vi "Do Calculation.vi"(8 "error in (no error)":errorcluster, 11 "CPU FFT Calculator in":refnum<class "CPU FFT Calculator.lvclass">) -> (0 "error out":errorcluster, 3 "CPU FFT Calculator out":refnum<class "CPU FFT Calculator.lvclass">)   [LabVIEW 2020, in "CPU FFT Calculator.lvlib" / "CPU FFT Calculator.lvclass"]
uses:
  CPU FFT Calculator.lvclass
  C:/Users/natan/Documents/G2CPU-Performance-Demo/Calculation Worker/Calculation Worker/Calculation Worker.lvclass
  C:/Program Files/National Instruments/LabVIEW 2026/vi.lib/ActorFramework/Actor/Actor.lvclass
  CPU FFT Calculator.lvclass/CPU FFT Calculator.ctl
  CPU Calculation Results.ctl
  <vilib>/ActorFramework/Actor/Actor.lvclass/Actor.ctl
  <vilib>/ActorFramework/Message Enqueuer/Message Enqueuer.lvclass/Message Enqueuer.ctl
  CPU FFT Calculator Messages/Process Calculation Results Msg/Process Calculation Results Msg.lvclass/Process Calculation Results Msg.ctl
  <vilib>/Analysis/2dsp.llb/Complex FFT.vi
  <vilib>/ActorFramework/Message Enqueuer/Init from Existing Queue.vi
  <vilib>/ActorFramework/Message Enqueuer/Enqueue.vi
  CPU FFT Calculator Messages/Process Calculation Results Msg/Process Calculation Results Msg.lvclass
  C:/Program Files/National Instruments/LabVIEW 2026/vi.lib/ActorFramework/Message/Message.lvclass
  CPU FFT Calculator Messages/Do Calculation Msg/Do Calculation Msg.lvclass
  CPU FFT Calculator Messages/Stop Calculation Msg/Stop Calculation Msg.lvclass
  <vilib>/ActorFramework/Message Priority Queue/Priority Enqueue.vi
  <vilib>/ActorFramework/Message Enqueuer/Message Enqueuer.lvclass
  <vilib>/Analysis/NI_AALPro.lvlib
  <vilib>/ActorFramework/Actor/Actor.lvclass
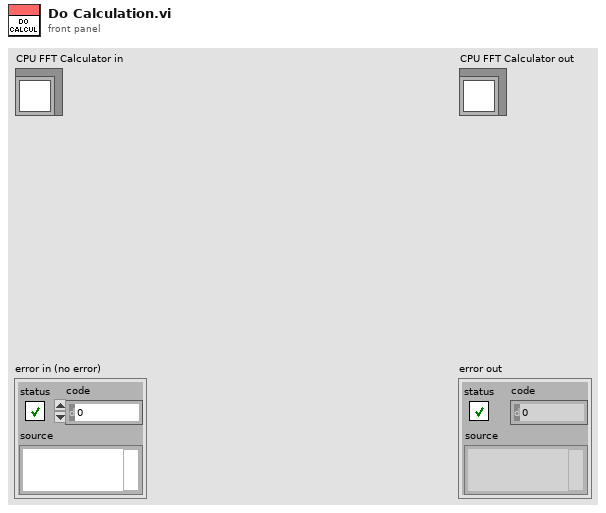
[diagram p1: front panel]
types:
  T1 = typedef "CPU FFT Calculator.lvlib/CPU FFT Calculator.lvclass/CPU Calculation Results.ctl" = cluster{"Result Array":sgl[], "Throughput Time":dbl, "FFT Time":dbl, "Buffer Size":i32}
  T2 = typedef "Data Source.lvlib/Data Source.lvclass/Data Source Buffer.ctl" = refnum<data-value>
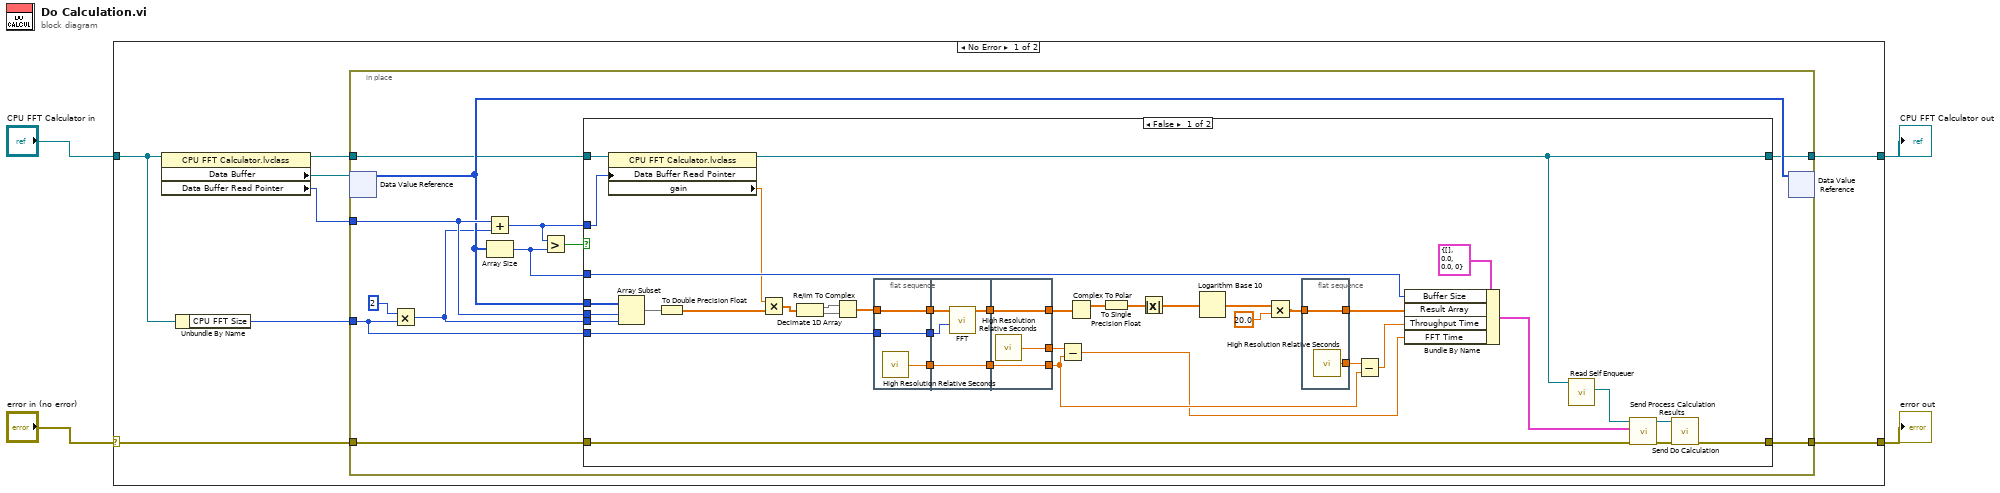
[diagram p0: block diagram]
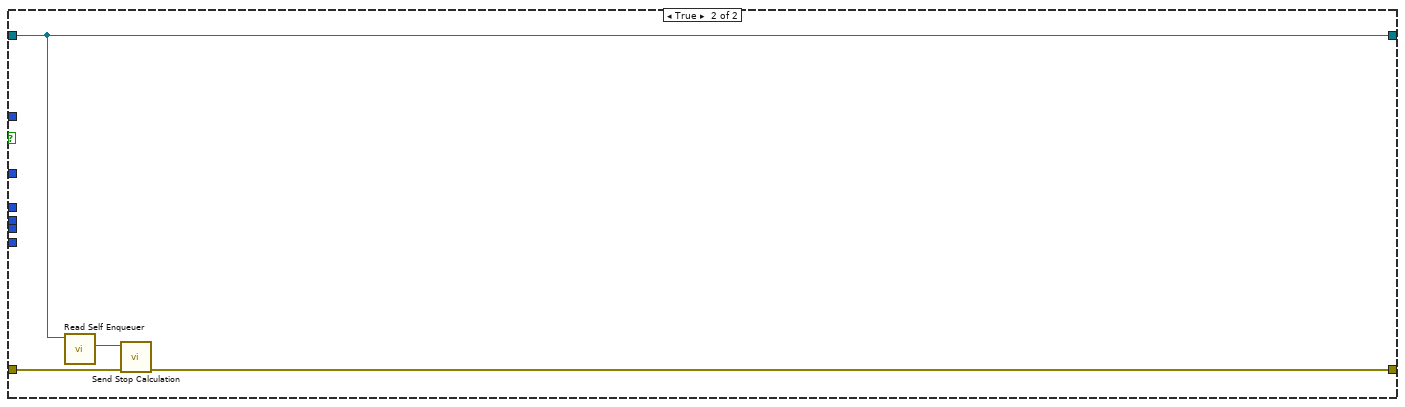
[diagram p2: hidden frame]
diagram:
  n1 = case shown="No Error" "error in (no error)" {
    selector: "error in (no error)" -> [w8 w82]
    tunnel: [w7 w82] -> w3
    tunnel: [w5 w81] -> w1
    tunnel: "CPU FFT Calculator in" -> [w12 w81]
    frame No Error {
      n2 = property class="CPU FFT Calculator.lvclass"(reference=w12) -> (reference out=w6:refnum<class "CPU FFT Calculator.lvclass">, "Data Buffer"=w11:T2, "Data Buffer Read Pointer"=w9:u64)  [unwired: 1 in, 1 out]
      n3 = Unbundle By Name(w12) -> ("CPU FFT Size"=w10:u64)
      n4 = in-place {
        in-place-border: w10 -> [w15]
        in-place-border: w9 -> [w24]
        in-place-border: w8 -> [w22]
        in-place-border: [w20] -> w7
        in-place-border: w6 -> [w19]
        in-place-border: [w17] -> w5
        n5 = in-place-dvr #1(w11) -> (w23:i16[])  [unwired: 1 out]
        n6 = Multiply(x=u64 2, y=w15) -> (x*y=w14:u64)
        n7 = Add(x=w24, y=w14) -> (x+y=w18:u64)
        n8 = Array Size(array=w23) -> (size(s)=w16:i32)
        n9 = Greater?(x=w18, y=w16) -> (0:w21:bool)
        n10 = case shown="False" w21 {
          tunnel: w24 -> [w51 _]
          tunnel: w14 -> [w50 _]
          tunnel: w23 -> [w46 _]
          tunnel: w22 -> [w38 w80]
          tunnel: [w37 w79] -> w20
          tunnel: w19 -> [w35 w77]
          tunnel: w18 -> [w34 _]
          tunnel: [w33 w77] -> w17
          tunnel: w16 -> [w32 _]
          tunnel: w15 -> [w31 _]
          frame False {
            n11 = property class="CPU FFT Calculator.lvclass"(reference=w35, "Data Buffer Read Pointer"=w34) -> (reference out=w33:refnum<class "CPU FFT Calculator.lvclass">, "gain"=w25:dbl)  [unwired: 1 in, 1 out]
            n12 = Array Subset(array=w46, index=w51, length=w50) -> (w53:i16[])
            n13 = To Double Precision Float(number=w53) -> (double precision float=w30:dbl[])
            n14 = Multiply(x=w25, y=w30) -> (x*y=w26:dbl[])
            n15 = Decimate 1D Array(w26) -> (w29:dbl[], w28:dbl[])
            n16 = Re/Im To Complex(1:w28, 2:w29) -> (0:w27:cdb[])
            n17 = flat-sequence {
              tunnel: w31 -> [w68]
              tunnel: w27 -> [w69]
              tunnel: [w69] -> w64
              tunnel: [w68] -> w63
              tunnel: [w67] -> w62
              tunnel: [w73] -> w61
              tunnel: w64 -> [w72]
              tunnel: w63 -> [w71]
              tunnel: w62 -> [w70]
              tunnel: [w70] -> w60
              tunnel: [w76] -> w54
              tunnel: w61 -> [w76]
              tunnel: [w75] -> w52
              tunnel: w60 -> [w74]
              tunnel: [w74] -> w47
              frame #0 {
                n18 = call <vilib>:"High Resolution Relative Seconds.vi"() -> ("relative seconds"=w67:dbl)
              }
              frame #1 {
                n19 = call-poly <vilib>:"FFT.vi"("FFT size"=w71, "X"=w72) -> ("FFT {X}"=w73:cdb[])  [unwired: 8 in, 1 out]
              }
              frame #2 {
                n20 = call <vilib>:"High Resolution Relative Seconds.vi"() -> ("relative seconds"=w75:dbl)
              }
            }
            n21 = Subtract(x=w52, y=w47) -> (x-y=w39:dbl)
            n22 = Complex To Polar(r * e^(i*theta)=w54) -> (r=w55:dbl[])  [unwired: 1 out]
            n23 = To Single Precision Float(number=w55) -> (single precision float=w56:sgl[])
            n24 = Absolute Value(x=w56) -> (abs(x)=w59:sgl[])
            n25 = Logarithm Base 10(1:w59) -> (0:w58:sgl[])
            n26 = Multiply(x=w58, y=sgl 20.0) -> (x*y=w49:sgl[])
            n27 = flat-sequence {
              tunnel: [w66] -> w41
              tunnel: w49 -> [w66]
              tunnel: [w65] -> w48
              frame #0 {
                n28 = call <vilib>:"High Resolution Relative Seconds.vi"() -> ("relative seconds"=w65:dbl)
              }
            }
            n29 = Subtract(x=w48, y=w47) -> (x-y=w40:dbl)
            n30 = Bundle By Name(cluster=T1 {"Result Array"=[], "Throughput Time"=0.0, "FFT Time"=0.0, "Buffer Size"=0} ("Calculation Results"), "Buffer Size"=w32, "Result Array"=w41, "Throughput Time"=w40, "FFT Time"=w39) -> (w45:T1)
            n31 = call <vilib>:"Read Self Enqueuer.vi"("Actor"=w33) -> ("Self Enqueuer"=w44:refnum<class "Message Enqueuer.lvclass">)  [unwired: 10 in]
            n32 = call "Send Process Calculation Results.vi"("error in (no error)"=w38, "Calculation Results"=w45, "Message Enqueuer"=w44) -> ("error out"=w36:errorcluster, "Message Enqueuer out"=w43:refnum<class "Message Enqueuer.lvclass">)  [unwired: 7 in]
            n33 = call "Send Do Calculation.vi"("error in (no error)"=w36, "Message Enqueuer"=w43) -> ("error out"=w37:errorcluster)  [unwired: 8 in, 1 out]
          }
          frame True {
            n34 = call <vilib>:"Read Self Enqueuer.vi"("Actor"=w77) -> ("Self Enqueuer"=w78:refnum<class "Message Enqueuer.lvclass">)  [unwired: 10 in]
            n35 = call "Send Stop Calculation.vi"("error in (no error)"=w80, "Message Enqueuer"=w78) -> ("error out"=w79:errorcluster)  [unwired: 8 in, 1 out]
          }
        }
        n36 = in-place-dvr #1(w23) -> ()  [unwired: 2 out]
      }
    }
    frame Error {
    }
  }
  "error out" <- w3
  "CPU FFT Calculator out" <- w1
